vi "Configure Sync Output.vi"(4 "Point Marker (4)":dbl=4.0, 5 "Sync Polarity (0: Normal)":i32(ring) items=["Normal", "Inverted"], 6 "Cycle Marker (2)":dbl=2.0, 7 "Sync Mode (0: Normal)":i32(ring) items=["Normal", "Carrier", "Marker"], 8 "error in (no error)":errorcluster, 9 "Channel (1: 1)":i32(ring)=1 items=["1"=1, "2"=2], 10 "Frequency Marker (500 Hz)":dbl=500.0, 11 "VISA resource name":refnum<visa-resource-name>) -> (0 "error out":errorcluster, 3 "VISA resource name out":refnum<visa-resource-name>)   [LabVIEW 2018, in "Agilent 3352X Series.lvlib"]
doc: "Enables output sync and configure behavior mode, polarity and markers for sync output signal."
uses:
  <instrlib>/Agilent 3352X Series/Agilent 3352X Series.lvlib
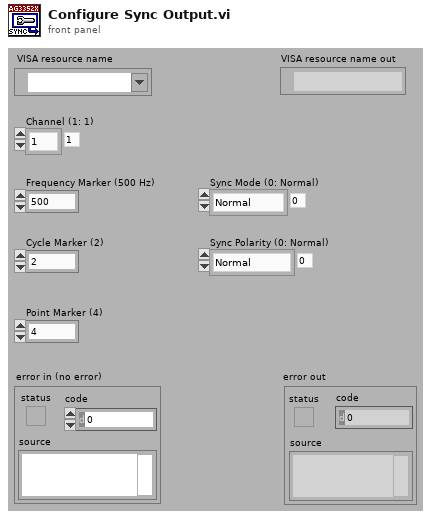
[diagram p1: front panel]
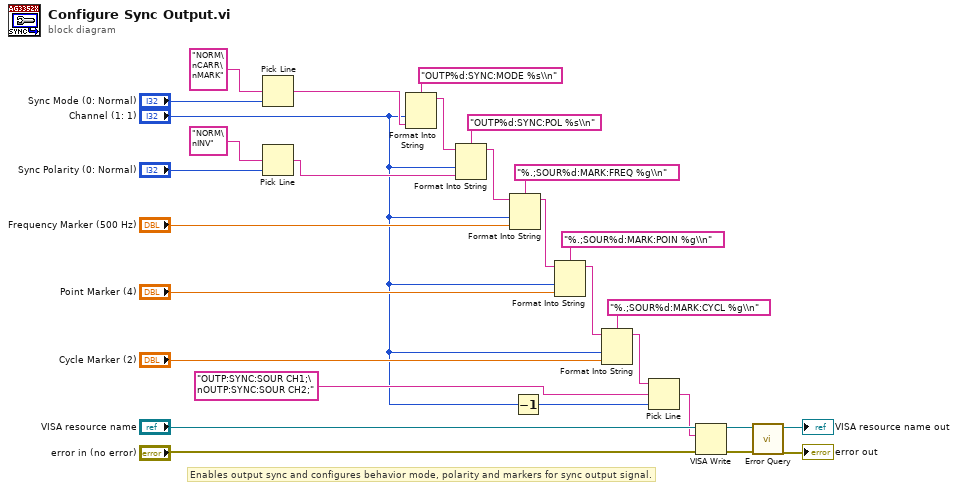
[diagram p0: block diagram]
diagram:
  # "Enables output sync and configures behavior mode, polarity and markers for sync output signal."
  n1 = Pick Line(multi-line string="NORM\nCARR\nMARK", line index="Sync Mode (0: Normal)") -> (output string=w18:string)  [unwired: 1 out]
  n2 = Pick Line(multi-line string="NORM\nINV", line index="Sync Polarity (0: Normal)") -> (output string=w15:string)  [unwired: 1 out]
  n3 = Format Into String(format string="OUTP%d:SYNC:MODE %s\\n", "Channel (1: 1)", w18) -> (resulting string=w28:string)  [unwired: 2 in, 1 out]
  n4 = Format Into String(format string="OUTP%d:SYNC:POL %s\\n", initial string=w28, "Channel (1: 1)", w15) -> (resulting string=w13:string)  [unwired: 1 in, 1 out]
  n5 = Format Into String(format string="%.;SOUR%d:MARK:FREQ %g\\n", initial string=w13, "Channel (1: 1)", "Frequency Marker (500 Hz)") -> (resulting string=w10:string)  [unwired: 1 in, 1 out]
  n6 = Decrement(x="Channel (1: 1)") -> (x-1=w1:i32)
  n7 = Format Into String(format string="%.;SOUR%d:MARK:POIN %g\\n", initial string=w10, "Channel (1: 1)", "Point Marker (4)") -> (resulting string=w9:string)  [unwired: 1 in, 1 out]
  n8 = Format Into String(format string="%.;SOUR%d:MARK:CYCL %g\\n", initial string=w9, "Channel (1: 1)", "Cycle Marker (2)") -> (resulting string=w7:string)  [unwired: 1 in, 1 out]
  n9 = Pick Line(string ("")=w7, multi-line string="OUTP:SYNC:SOUR CH1;\nOUTP:SYNC:SOUR CH2;", line index=w1) -> (output string=w8:string)
  n10 = VISA Write(VISA resource name="VISA resource name", write buffer=w8, error in (no error)="error in (no error)") -> (VISA resource name out=w24:refnum<visa-resource-name>, error out=w23:errorcluster)  [unwired: 1 out]
  n11 = call <instrlib>:"Error Query.vi"("error in (no error)"=w23, "VISA resource name"=w24) -> ("error out"=→"error out":errorcluster, "VISA resource name out"=→"VISA resource name out":refnum<visa-resource-name>)  [unwired: 8 out]
